vi "Equals Data Type.vi"(8 "error in":errorcluster, 10 "Data Type":T1=1 items=["BOOLEAN"=1, "INTEGER8"=2, "INTEGER16"=3, "INTEGER32"=4, "UNSIGNED8"=5, "UNSIGNED16"=6, "UNSIGNED32"=7, "REAL32"=8, "VISIBLE_STRING"=9, "OCTET_STRING"=10, "UNICODE_STRING"=11, "TIME_OF_DAY"=12, "TIME_DIFFERENCE"=13, "RESERVED1"=14, "DOMAIN"=15, "INTEGER24"=16, "REAL64"=17, "INTEGER40"=18, "INTEGER48"=19, "INTEGER56"=20, "INTEGER64"=21, "UNSIGNED24"=22, "RESERVED2"=23, "UNSIGNED40"=24, "UNSIGNED48"=25, "UNSIGNED56"=26, "UNSIGNED64"=27, "RESERVED3"=28, "RESERVED4"=29, "RESERVED5"=30, "RESERVED6"=31, "PDO_COMMUNICATION_PARAMETER"=32, "PDO_MAPPING"=33, "SDO_PARAMETER"=34, "IDENTITY"=35, "RESERVED7"=36], 11 "Sub Obj in":refnum<class "Sub Object.lvclass">) -> (0 "error out":errorcluster, 2 "Equal":bool, 3 "Sub Obj out":refnum<class "Sub Object.lvclass">)   [LabVIEW 2020, in "CANopen.lvlib" / "Sub Object.lvclass"]
uses:
  Sub Object.lvclass
  Sub Object.lvclass/Sub Object.ctl
  Typedefs/Data Type.ctl
  CANopen.lvlib
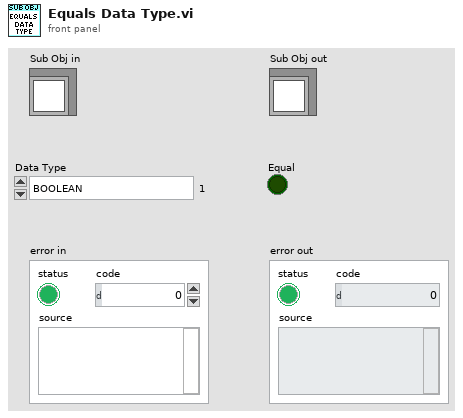
[diagram p1: front panel]
types:
  T1 = typedef "CANopen.lvlib/Data Type.ctl" = u16
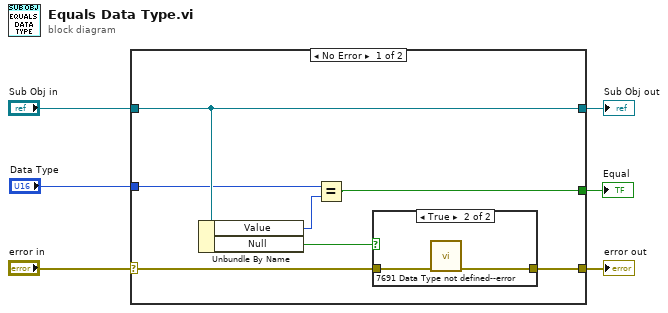
[diagram p0: block diagram]
diagram:
  n1 = case shown="No Error" "error in" {
    selector: "error in" -> [w11 w18]
    tunnel: [w10 w18] -> w3
    tunnel: [w13 w17] -> w5
    tunnel: "Sub Obj in" -> [w13 w17]
    tunnel: "Data Type" -> [w8 _]
    tunnel: [w7 _] -> w1
    frame No Error {
      n2 = Unbundle By Name(w13) -> ("Value"=w9:T1, "Null"=w12:bool)
      n3 = Equal?(x=w8, y=w9) -> (x = y?=w7:bool)
      n4 = case shown="True" w12 {
        tunnel: w11 -> [w14 w16]
        tunnel: [w14 w15] -> w10
        frame False {
        }
        frame True {
          n5 = call "7691 Data Type not defined--error.vi"("error in"=w16) -> ("error out"=w15:errorcluster)  [unwired: 9 in, 1 out]
        }
      }
    }
    frame Error {
    }
  }
  "Sub Obj out" <- w5
  "error out" <- w3
  "Equal" <- w1
